vi "Optim joy manipulator.vi"(8 "device index":i32=7) -> (0 "error out":errorcluster, 1 "Refnum out":refnum<k1>, 2 "output cluster":T1, 5 "POV":bool, 7 "axis info":T4, 10 "wysylanie":bool)   [LabVIEW 2015]
uses:
  wyj manip.ctl
  <vilib>/Utility/inputDevices.llb/joystickAcquire.vi
panel:
  out "direction info":T2
  out "button info":T3
  out "Cluster":T5
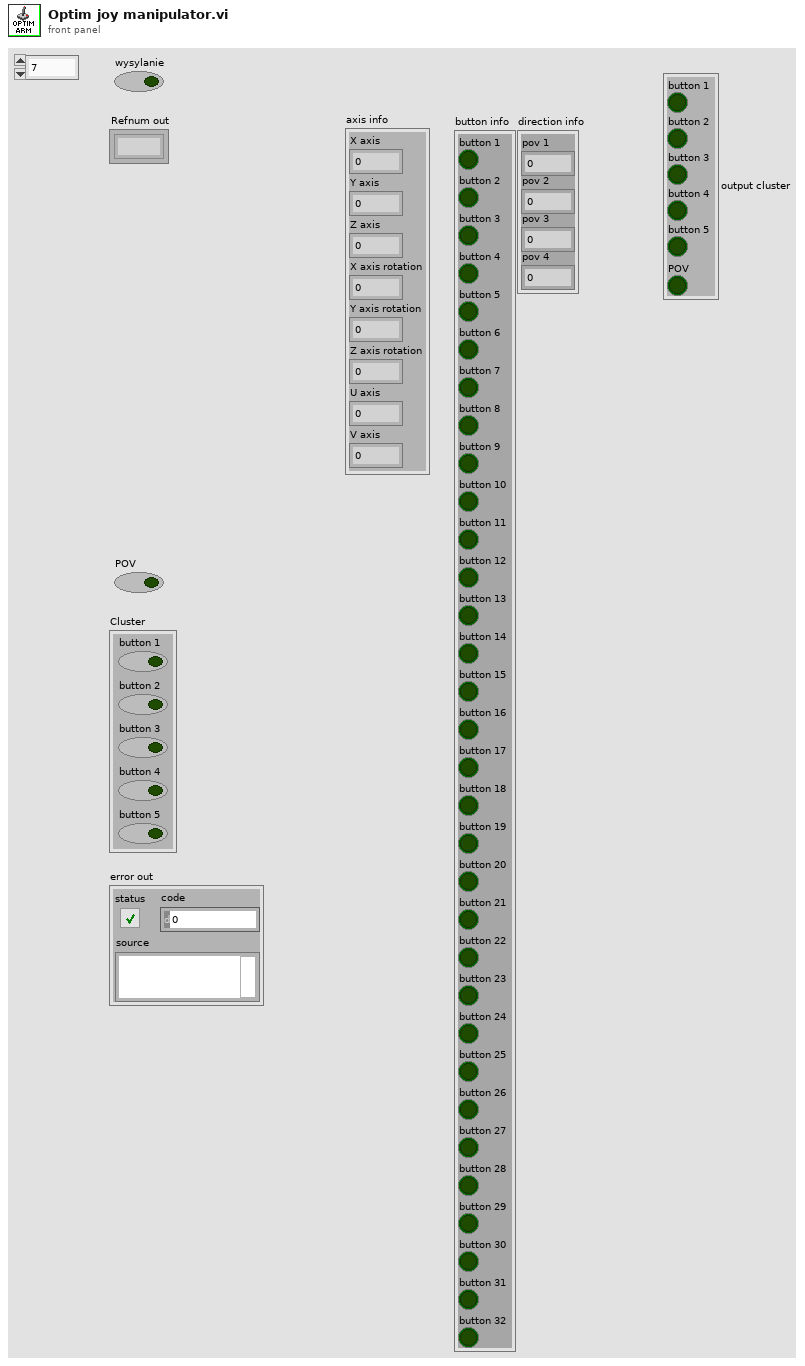
[diagram p1: front panel]
types:
  T1 = typedef "wyj manip.ctl" = cluster{"button 1":bool, "button 2":bool, "button 3":bool, "button 4":bool, "button 5":bool, "POV":bool}
  T2 = cluster{"pov 1":i32, "pov 2":i32, "pov 3":i32, "pov 4":i32}
  T3 = cluster{"button 1":bool, "button 2":bool, "button 3":bool, "button 4":bool, "button 5":bool, "button 6":bool, "button 7":bool, "button 8":bool, "button 9":bool, "button 10":bool, "button 11":bool, "button 12":bool, "button 13":bool, "button 14":bool, "button 15":bool, "button 16":bool, "button 17":bool, "button 18":bool, "button 19":bool, "button 20":bool, "button 21":bool, "button 22":bool, "button 23":bool, "button 24":bool, "button 25":bool, "button 26":bool, "button 27":bool, "button 28":bool, "button 29":bool, "button 30":bool, "button 31":bool, "button 32":bool}
  T4 = cluster{"X axis":i32, "Y axis":i32, "Z axis":i32, "X axis rotation":i32, "Y axis rotation":i32, "Z axis rotation":i32, "U axis":i32, "V axis":i32}
  T5 = cluster{"button 1":bool, "button 2":bool, "button 3":bool, "button 4":bool, "button 5":bool}
  T6 = cluster{"button 1":bool, "button 2":bool, "button 3":bool, "button 4":bool, "button 5":bool, bool}
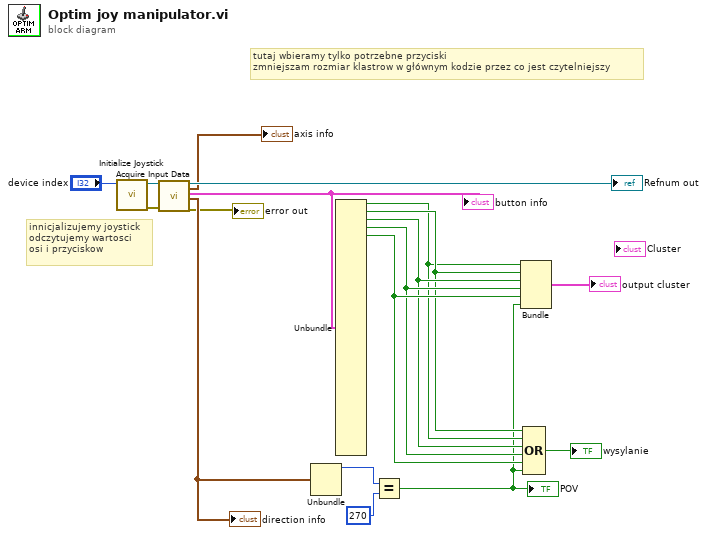
[diagram p0: block diagram]
diagram:
  # "innicjalizujemy joystick\nodczytujemy wartosci \nosi i przyciskow"
  # "tutaj wbieramy tylko potrzebne przyciski \nzmniejszam rozmiar klastrow w głównym kodzie przez co jest czytelniejszy"
  n1 = call <vilib>:"Initialize Joystick.vi"("device index"="device index") -> ("error out"=w11:errorcluster, "device ID"=w3:refnum<k1>)  [unwired: 9 in]
  n2 = call-poly <vilib>:"Acquire Input Data.vi"("device ID"=w3, "error in (no error)"=w11) -> ("device ID"=→"Refnum out":refnum<k1>, "axis info"=→"axis info":T4, "button info"=w5:T3, "direction info"=w12:T2, "error out"=→"error out":errorcluster)  [unwired: 13 in]
  "button info" <- w5
  "direction info" <- w12
  n3 = Unbundle(w12) -> ("pov 1"=w6:i32)  [unwired: 3 out]
  n4 = Unbundle(w5) -> ("button 1"=w14:bool, "button 2"=w15:bool, "button 3"=w16:bool, "button 4"=w17:bool, "button 5"=w18:bool)  [unwired: 27 out]
  n5 = Equal?(x=w6, y=270) -> (x = y?=w2:bool)
  "POV" <- w2
  n6 = Bundle("button 1"=w14, "button 2"=w15, "button 3"=w16, "button 4"=w17, "button 5"=w18, w2) -> (→"output cluster":T6)  [unwired: 1 in]
  n7 = Compound Arithmetic op=OR(w15, w14, w16, w17, w18, w2) -> (→"wysylanie":bool)
